vi "获取配置文件.vi"(8 "错误输入":errorcluster) -> (0 "错误输出":errorcluster, 1 "路径输出":path, 3 "数组":string[](array[string]))   [LabVIEW 2021]
panel:
  out "文件名":string[](array[string])
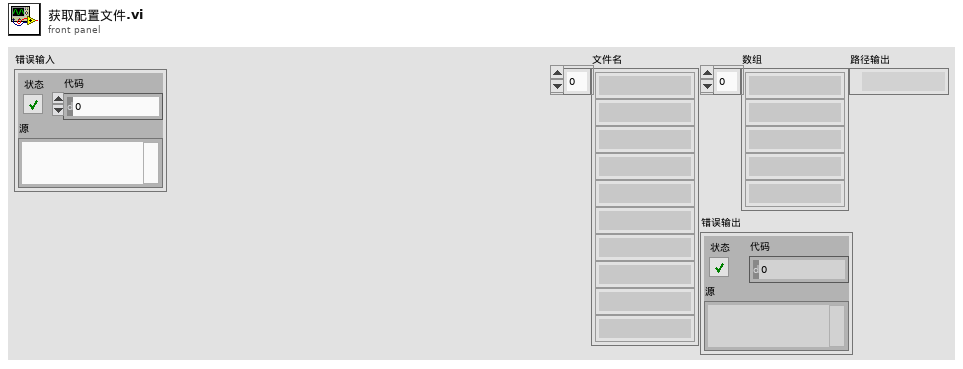
[diagram p1: front panel]
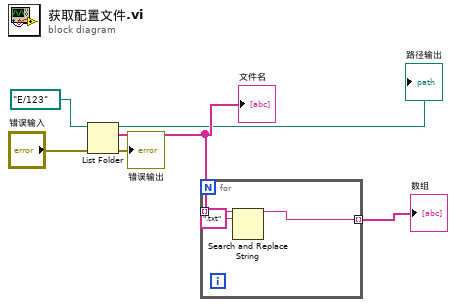
[diagram p0: block diagram]
diagram:
  n1 = List Folder(path=path "E:/123" ("路径"), error in="错误输入") -> (path out=→"路径输出":path, filenames=w6:string[], error out=→"错误输出":errorcluster)  [unwired: 2 in, 1 out]
  "文件名" <- w6
  n2 = for {
    tunnel: w6 -> [w9] mode=indexing
    tunnel: [w7] -> w5 mode=indexing
    n3 = Search and Replace String(input string=w9, search string=".txt" ("搜索字符串")) -> (result string=w7:string)  [unwired: 6 in, 3 out]
  }
  "数组" <- w5
